vi "prepare_press.vi"(10 "压力设定值（KPa）":dbl[](array[numeric])=[100.0, 15000.0], 11 "CONST820":refnum<visa-resource-name>="COM3") -> ()   [LabVIEW 2017]
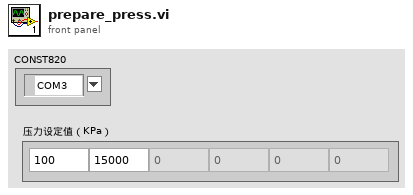
[diagram p1: front panel]
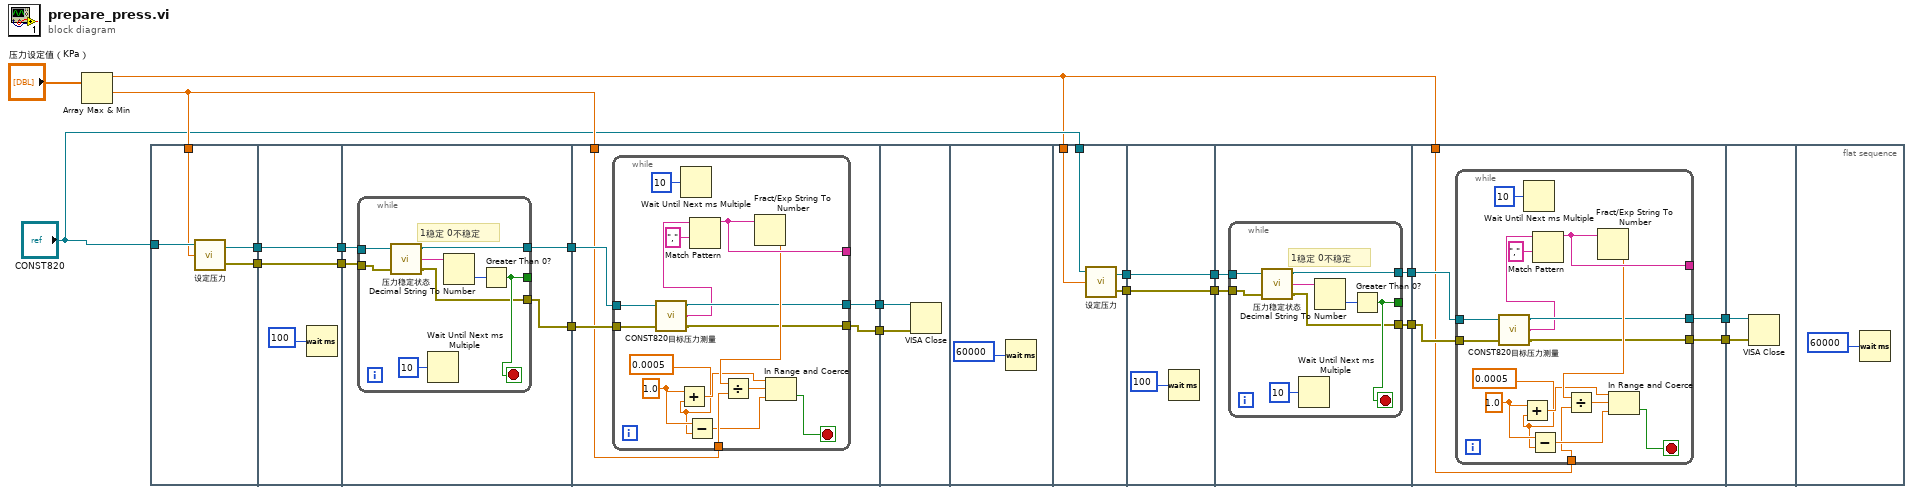
[diagram p0: block diagram]
diagram:
  n1 = Array Max & Min(array="压力设定值（KPa）") -> (max value=w3:dbl, min value=w13:dbl)  [unwired: 2 out]
  n2 = flat-sequence {
    tunnel: "CONST820" -> [w24]
    tunnel: w13 -> [w23]
    tunnel: [w22] -> w18
    tunnel: [w21] -> w16
    tunnel: [w26] -> w19
    tunnel: w18 -> [w26]
    tunnel: [w25] -> w17
    tunnel: w16 -> [w25]
    tunnel: w19 -> [w31]
    tunnel: w17 -> [w30]
    tunnel: [w29] -> w15
    tunnel: [w28] -> w14
    tunnel: w15 -> [w44]
    tunnel: w14 -> [w43]
    tunnel: w13 -> [w42]
    tunnel: [w41] -> w12
    tunnel: [w40] -> w11
    tunnel: w12 -> [w62]
    tunnel: w11 -> [w61]
    tunnel: "CONST820" -> [w67]
    tunnel: w3 -> [w66]
    tunnel: [w65] -> w9
    tunnel: [w64] -> w8
    tunnel: w9 -> [w70]
    tunnel: w8 -> [w69]
    tunnel: [w70] -> w7
    tunnel: [w69] -> w6
    tunnel: w7 -> [w74]
    tunnel: w6 -> [w73]
    tunnel: [w72] -> w5
    tunnel: [w71] -> w4
    tunnel: w5 -> [w87]
    tunnel: w4 -> [w86]
    tunnel: w3 -> [w85]
    tunnel: [w84] -> w2
    tunnel: [w83] -> w1
    tunnel: w2 -> [w105]
    tunnel: w1 -> [w104]
    frame #0 {
      n3 = call "设定压力.vi"("设定"=w23, "VISA resource name"=w24) -> ("错误输出"=w21:errorcluster, "VISA资源名称输出"=w22:refnum<visa-resource-name>)  [unwired: 1 in]
    }
    frame #1 {
      n4 = Wait (ms)(milliseconds to wait=u32 100 ("毫秒计时值")) -> ()  [unwired: 1 out]
    }
    frame #2 {
      n5 = while {
        tunnel: w31 -> [w36]
        tunnel: w30 -> [w35]
        tunnel: [w38] -> _
        tunnel: [w34] -> w29
        tunnel: [w33] -> w28
        stop <- w38 stop-if-true
        # "1稳定 0不稳定"
        n6 = call "压力稳定状态.vi"("error in (no error) 2"=w35, "VISA resource name"=w36) -> ("错误输出"=w33:errorcluster, "状态(1稳定)"=w32:string, "VISA资源名称输出"=w34:refnum<visa-resource-name>)  [unwired: 1 in]
        n7 = Wait Until Next ms Multiple(millisecond multiple=u32 10 ("毫秒倍数")) -> ()  [unwired: 1 out]
        n8 = Decimal String To Number(string=w32) -> (number=w39:i32)  [unwired: 2 in, 1 out]
        n9 = Greater Than 0?(x=w39) -> (x > 0?=w38:bool)
      }
    }
    frame #3 {
      n10 = while {
        tunnel: w44 -> [w53]
        tunnel: w43 -> [w46]
        tunnel: [w52] -> w41
        tunnel: [w50] -> w40
        tunnel: [w59] -> _
        tunnel: w42 -> [w57]
        stop <- w55 stop-if-true
        w45 = 0.0005
        w48 = 1.0 ("上限")
        n11 = call "CONST820目标压力测量.vi"("error in (no error) 2"=w46, "VISA resource name"=w53) -> ("错误输出"=w50:errorcluster, "目标压力值"=w51:string, "VISA资源名称输出"=w52:refnum<visa-resource-name>)  [unwired: 1 in]
        n12 = Add(x=w48, y=w45) -> (x+y=w49:dbl)
        n13 = Wait Until Next ms Multiple(millisecond multiple=u32 10 ("毫秒倍数")) -> ()  [unwired: 1 out]
        n14 = Subtract(x=w48, y=w45) -> (x-y=w47:dbl)
        n15 = Match Pattern(string=w51, regular expression="," ("正则表达式")) -> (before substring=w59:string)  [unwired: 1 in, 3 out]
        n16 = Fract/Exp String To Number(string=w59) -> (number=w58:dbl)  [unwired: 3 in, 1 out]
        n17 = Divide(x=w58, y=w57) -> (x/y=w56:dbl)
        n18 = In Range and Coerce(upper limit=w49, x=w56, lower limit=w47) -> (In Range?=w55:bool)  [unwired: 1 out]
      }
    }
    frame #4 {
      n19 = VISA Close(VISA resource name=w62, error in (no error)=w61) -> ()  [unwired: 1 out]
    }
    frame #5 {
      n20 = Wait (ms)(milliseconds to wait=u32 60000 ("毫秒计时值")) -> ()  [unwired: 1 out]
    }
    frame #6 {
      n21 = call "设定压力.vi"("设定"=w66, "VISA resource name"=w67) -> ("错误输出"=w64:errorcluster, "VISA资源名称输出"=w65:refnum<visa-resource-name>)  [unwired: 1 in]
    }
    frame #7 {
      n22 = Wait (ms)(milliseconds to wait=u32 100 ("毫秒计时值")) -> ()  [unwired: 1 out]
    }
    frame #8 {
      n23 = while {
        tunnel: w74 -> [w79]
        tunnel: w73 -> [w78]
        tunnel: [w81] -> _
        tunnel: [w77] -> w72
        tunnel: [w76] -> w71
        stop <- w81 stop-if-true
        # "1稳定 0不稳定"
        n24 = call "压力稳定状态.vi"("error in (no error) 2"=w78, "VISA resource name"=w79) -> ("错误输出"=w76:errorcluster, "状态(1稳定)"=w75:string, "VISA资源名称输出"=w77:refnum<visa-resource-name>)  [unwired: 1 in]
        n25 = Wait Until Next ms Multiple(millisecond multiple=u32 10 ("毫秒倍数")) -> ()  [unwired: 1 out]
        n26 = Decimal String To Number(string=w75) -> (number=w82:i32)  [unwired: 2 in, 1 out]
        n27 = Greater Than 0?(x=w82) -> (x > 0?=w81:bool)
      }
    }
    frame #9 {
      n28 = while {
        tunnel: w87 -> [w97]
        tunnel: w86 -> [w90]
        tunnel: [w96] -> w84
        tunnel: [w94] -> w83
        tunnel: [w102] -> _
        tunnel: w85 -> [w88]
        stop <- w99 stop-if-true
        w89 = 0.0005
        w92 = 1.0 ("上限")
        n29 = call "CONST820目标压力测量.vi"("error in (no error) 2"=w90, "VISA resource name"=w97) -> ("错误输出"=w94:errorcluster, "目标压力值"=w95:string, "VISA资源名称输出"=w96:refnum<visa-resource-name>)  [unwired: 1 in]
        n30 = Add(x=w92, y=w89) -> (x+y=w93:dbl)
        n31 = Wait Until Next ms Multiple(millisecond multiple=u32 10 ("毫秒倍数")) -> ()  [unwired: 1 out]
        n32 = Subtract(x=w92, y=w89) -> (x-y=w91:dbl)
        n33 = Match Pattern(string=w95, regular expression="," ("正则表达式")) -> (before substring=w102:string)  [unwired: 1 in, 3 out]
        n34 = Fract/Exp String To Number(string=w102) -> (number=w101:dbl)  [unwired: 3 in, 1 out]
        n35 = Divide(x=w101, y=w88) -> (x/y=w100:dbl)
        n36 = In Range and Coerce(upper limit=w93, x=w100, lower limit=w91) -> (In Range?=w99:bool)  [unwired: 1 out]
      }
    }
    frame #10 {
      n37 = VISA Close(VISA resource name=w105, error in (no error)=w104) -> ()  [unwired: 1 out]
    }
    frame #11 {
      n38 = Wait (ms)(milliseconds to wait=u32 60000 ("毫秒计时值")) -> ()  [unwired: 1 out]
    }
  }
